vi "Add Tag.vi"(9 "TagSet":T1, 11 "Series in":refnum<class "Series.lvclass">) -> (3 "Series out":refnum<class "Series.lvclass">)   [LabVIEW 2018, in "InfluxDB Client.lvlib" / "Series.lvclass"]
uses:
  Series.lvclass
  Controls/TagSet.ctl
  Series.lvclass/Series.ctl
  InfluxDB Client.lvlib
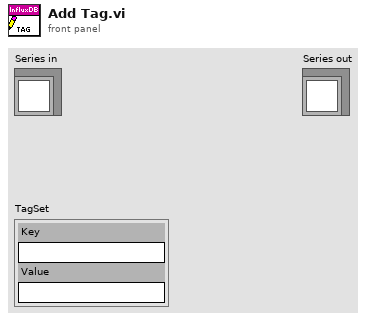
[diagram p1: front panel]
types:
  T1 = typedef "InfluxDB Client.lvlib/TagSet.ctl" = cluster{"Key":string, "Value":string}
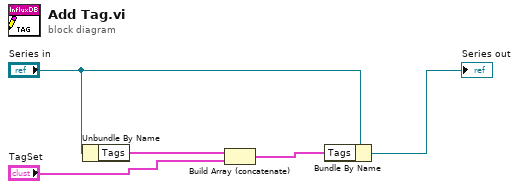
[diagram p0: block diagram]
diagram:
  n1 = Unbundle By Name("Series in") -> ("Tags"=w3:T1[])
  n2 = Build Array (concatenate)(w3, "TagSet") -> (w2:T1[])
  n3 = Bundle By Name(cluster="Series in", "Tags"=w2) -> (→"Series out":refnum<class "Series.lvclass">)
